vi "Get Connections - NPin MConn.vi"(8 "error in":errorcluster, 9 "site":i32=-1, 10 "pin or relay names":string[](array[string]), 11 "session reservation in":refnum<class "Session Reservation.lvclass">) -> (0 "error out":errorcluster, 2 "connections":T1[](array[typedef]), 3 "session reservation out":refnum<class "Session Reservation.lvclass">)   [LabVIEW 2020, in "MeasurementLink niDCPower.lvlib"]
doc: "Gets the NI-DCPower connection information for the given <b>pin or relay names</b> and <b>site</b>. If the <b>pin or relay names</b> input is unwired, the connection information for all pins for the given <b>site</b> will be returned. If the <b>site</b> input is unwired, the connection information for the given <b>pin or relay names</b> for all sites will be returned. If both the <b>pin or relay names</b> and <b>site</b> inputs are unwired, the connection information for all pins and all sites will be returned.\n\nIf you have not called <b>Create Sessions.vi</b> prior to calling this VI, the connection information will be returned with the correct information but will have an invalid session."
uses:
  MeasurementLink niDCPower.lvlib
  MeasurementLink Session Management/Session Reservation/Session Reservation.lvclass
  Connection with Session.ctl
  MeasurementLink Session Management/Session Reservation/Connection.ctl
  Instrument/Instrument.lvclass
  C:/dev/measurementlink-labview/Source/Runtime/MeasurementLink Instrument/IInstrument/IInstrument.lvclass
  1016b550-acf3-415d-ab7a-971f7ba5cd11.vi
  MeasurementLink Session Management/Session Reservation/Get Connections Impl.vi
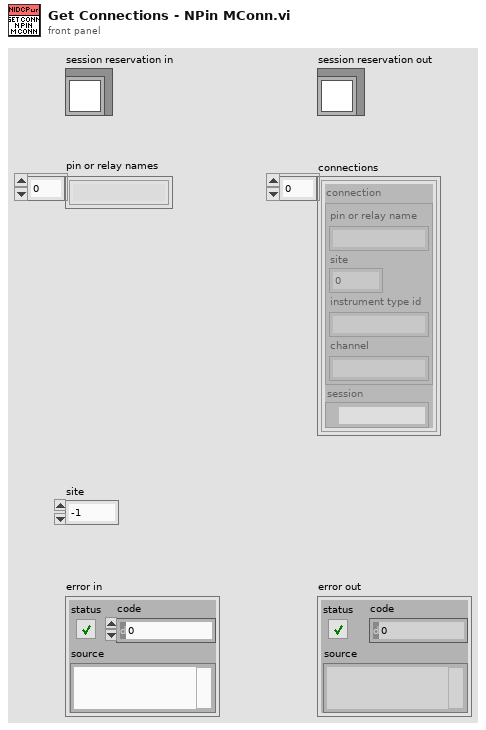
[diagram p1: front panel]
types:
  T1 = typedef "MeasurementLink niDCPower.lvlib/Connection with Session.ctl" = cluster{"connection":T2, "session":refnum<k15>}
  T2 = typedef "MeasurementLink Session Management.lvlib/Session Reservation.lvclass/Connection.ctl" = cluster{"pin or relay name":string, "site":i32, "instrument type id":string, "channel":string}
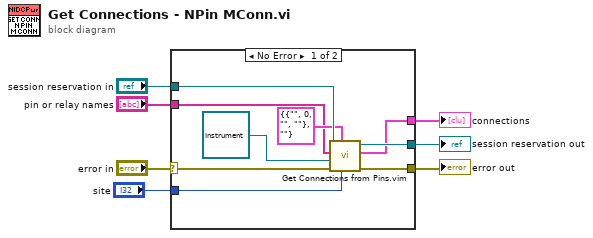
[diagram p0: block diagram]
diagram:
  n1 = case shown="No Error" "error in" {
    selector: "error in" -> [w9 w17]
    tunnel: "session reservation in" -> [w13 w18]
    tunnel: "pin or relay names" -> [w10 _]
    tunnel: [w14 w17] -> w4
    tunnel: [w16 w18] -> w3
    tunnel: [w15 _] -> w2
    tunnel: "site" -> [w12 _]
    frame No Error {
      n2 = call "Get Connections from Pins.vim"("site"=w12, "connection type"=T1 {"connection"={"pin or relay name"="", "site"=0, "instrument type id"="", "channel"=""}, "session"=""} ("niDCPower connection"), "error in"=w9, "instrument"=refnum<class "Instrument.lvclass"> refnum ("MeasurementLink niDCPower.lvlib:Instrument.lvclass"), "pin or relay names"=w10, "session reservation in"=w13) -> ("error out"=w14:errorcluster, "connections"=w15:T1[], "session reservation out"=w16:refnum<class "Session Reservation.lvclass">)  [unwired: 3 in]
    }
    frame Error {
    }
  }
  "error out" <- w4
  "session reservation out" <- w3
  "connections" <- w2
